vi "WriteReceiverState.vi"(8 "error in (no error)":errorcluster, 10 "tactic":T1, 11 "PrimaryAttackerRole in":refnum<class "PrimaryAttackerRole.lvclass">) -> (0 "error out":errorcluster, 3 "PrimaryAttackerRole out":refnum<class "PrimaryAttackerRole.lvclass">)   [LabVIEW 2023, in "PrimaryAttackerRole.lvclass"]
uses:
  PrimaryAttackerRole.lvclass
  C:/Users/ebert/Documents/codes/SSL/repo/SSL_AI/NewSTP/NewRoles/Role_v2_class/Role_v2.lvclass
  Robot_class/tactics.ctl
  PassTactic_class/PassTactic.lvclass
  C:/Users/ebert/Documents/codes/SSL/repo/SSL_AI/NewSTP/NewTactics/Tactic_v2_class/Tactic_v2.lvclass
  PrimaryAttackerRole_states.ctl
  NewSTP/NewRoles/Role_v2_class/Role_v2.lvclass/Role_v2.ctl
  NewSTP/NewRoles/Role_v2_class/Read Tactics.vi
  NewSTP/NewRoles/Role_v2_class/Write Tactics.vi
  NewSTP/NewTactics/Tactic_v2_class/Tactic_v2.lvclass
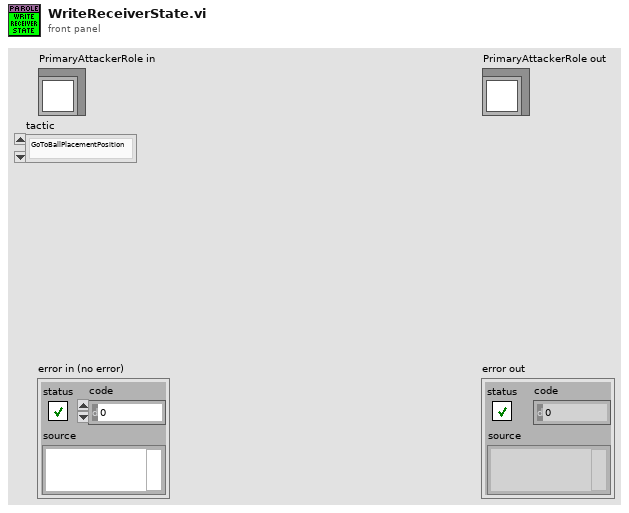
[diagram p1: front panel]
types:
  T1 = typedef "tactics.ctl" = enum16{"GoToBallPlacementPosition", "PlaceBall", "GoToBallPlacement", "5Robots", "BallPlacementEnemy", "ReceivePassInFuturePoint", "Roller", "PrepareRollToPassRollerGoTo", "PrepareRollToPassReceiverGoTo", "WaitRoll", "PositionToRoll", "PenaltyAttacker", "PassObserver", "PenaltyDefense", "TableReceiverTactic", "Test", "DefendGoal", "Marker", "FollowAttacker", "DefendArea", "Shoot", "AttackerAimGoal", "AttackerBallOutOfField", "AttackerBlock", "AttackerStop", "Duelist", "Halt", "ZigZag", "GoTo", "Timeout", "KickToBestRobot", "KickToPassReceiver", "PositionToReceivePass", "WaitPass"}
  T2 = typedef "PrimaryAttackerRole.lvclass/PrimaryAttackerRole_states.ctl" = enum16{"Intercept", "Shoot", "Pass"}
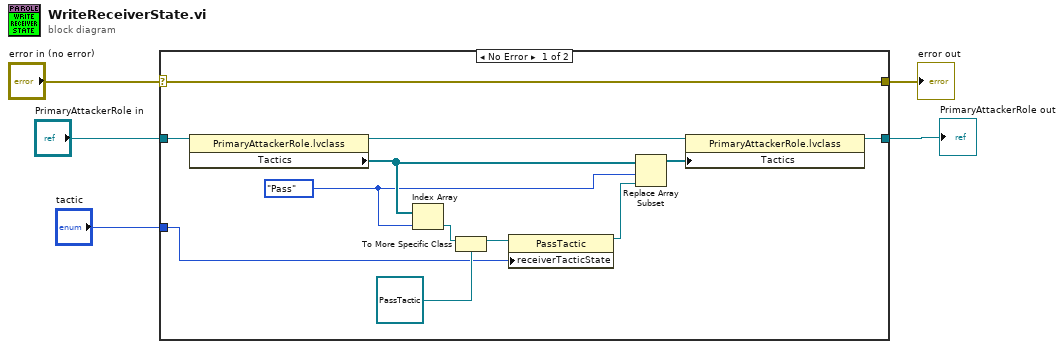
[diagram p0: block diagram]
diagram:
  n1 = case shown="No Error" "error in (no error)" {
    selector: "error in (no error)" -> [w17 w18]
    tunnel: [w17 w18] -> w4
    tunnel: [w6 w19] -> w2
    tunnel: "PrimaryAttackerRole in" -> [w16 w19]
    tunnel: "tactic" -> [w12 _]
    frame No Error {
      w10 = PrimaryAttackerRole_states."Pass" ("Enum")
      n2 = property class="PrimaryAttackerRole.lvclass"(reference=w16) -> (reference out=w7:refnum<class "PrimaryAttackerRole.lvclass">, "Tactics"=w11:refnum<class "Tactic_v2.lvclass">[])  [unwired: 1 in, 1 out]
      n3 = Index Array(array=w11, index=w10) -> (element=w14:refnum<class "Tactic_v2.lvclass">)
      n4 = To More Specific Class(target class=refnum<class "PassTactic.lvclass"> refnum ("PassTactic"), reference=w14) -> (specific class reference=w13:refnum<class "PassTactic.lvclass">)  [unwired: 1 in, 1 out]
      n5 = property class="PassTactic"(reference=w13, "receiverTacticState "=w12) -> (reference out=w9:refnum<class "PassTactic.lvclass">)  [unwired: 1 in, 1 out]
      n6 = Replace Array Subset(array=w11, new element=w9, index=w10) -> (w8:refnum<class "Tactic_v2.lvclass">[])
      n7 = property class="PrimaryAttackerRole.lvclass"(reference=w7, "Tactics"=w8) -> (reference out=w6:refnum<class "PrimaryAttackerRole.lvclass">)  [unwired: 1 in, 1 out]
    }
    frame Error {
    }
  }
  "error out" <- w4
  "PrimaryAttackerRole out" <- w2
